vi "Default Instrument Setup.vi"(8 "error in (no error)":errorcluster, 11 "VISA resource name":refnum<visa-resource-name>) -> (0 "error out":errorcluster, 3 "VISA resource name out":refnum<visa-resource-name>)   [LabVIEW 2013, in "Tektronix DPO MSO 2000 4000 Series.lvlib"]
doc: "This Utility VI sends a default command string to the instrument whenever a new VISA session is opened, or the instrument is reset. Use this VI as a subVI for the <B>Initialize</B> and <B>Reset</B> VIs. Altering this VI could cause these two VIs to operate incorrectly."
uses:
  Tektronix DPO MSO 2000 4000 Series.lvlib
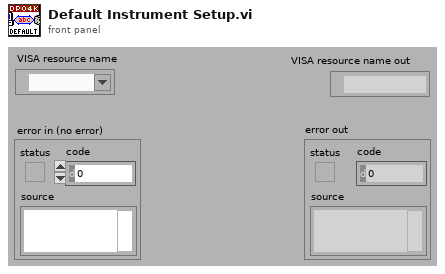
[diagram p1: front panel]
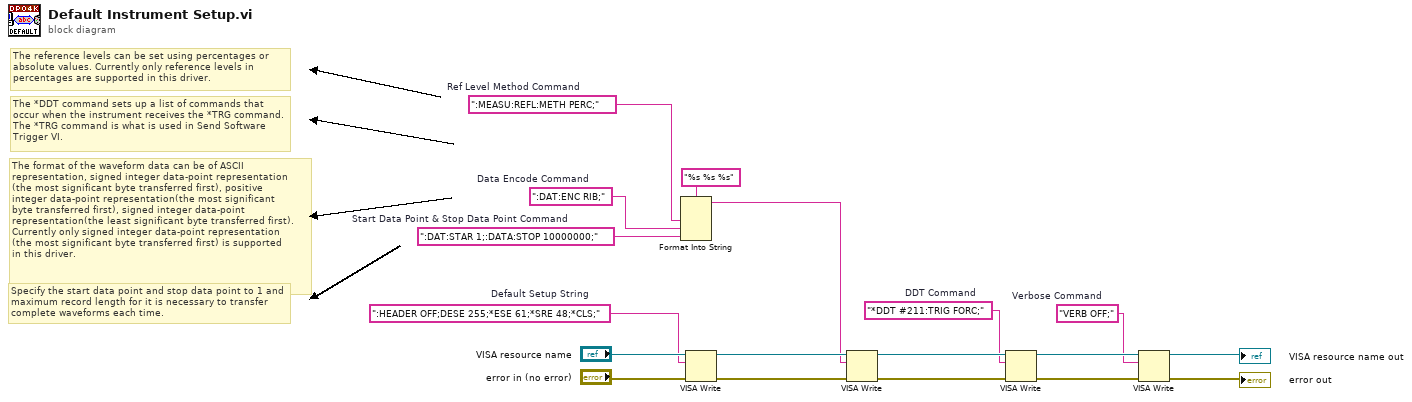
[diagram p0: block diagram]
diagram:
  w1 = "VERB OFF;"  # Verbose Command
  w6 = "*DDT #211:TRIG FORC;"  # DDT Command
  w10 = ":DAT:ENC RIB;"  # Data Encode Command
  w15 = ":MEASU:REFL:METH PERC;"  # Ref Level Method Command
  w9 = ":DAT:STAR 1;:DATA:STOP 10000000;"  # Start Data Point & Stop Data Point Command
  w16 = ":HEADER OFF;DESE 255;*ESE 61;*SRE 48;*CLS;"  # Default Setup String
  # "Specify the start data point and stop data point to 1 and maximum record length for it is necessary to transfer complete waveforms each time."
  # "The format of the waveform data can be of ASCII\nrepresentation, signed integer data-point representation\n(the most significant byte transferred first), positive \ninteger data-point representation(the most significant \nbyte transferred first), signed integer data-point \nrepresentation(the least significant byte transferred first).\nCurrently only signed integer data-point representation\n(the most significant byte transferred first) is supported\nin this driver."
  # "The reference levels can be set using percentages or absolute values. Currently only reference levels in \npercentages are supported in this driver."
  # "The *DDT command sets up a list of commands that occur when the instrument receives the *TRG command.  \nThe *TRG command is what is used in Send Software Trigger VI."
  n1 = Format Into String(format string="%s %s %s", w15, w10, w9) -> (resulting string=w12:string)  [unwired: 2 in, 1 out]
  n2 = VISA Write(VISA resource name="VISA resource name", write buffer=w16, error in (no error)="error in (no error)") -> (VISA resource name out=w14:refnum<visa-resource-name>, error out=w13:errorcluster)  [unwired: 1 out]
  n3 = VISA Write(VISA resource name=w14, write buffer=w12, error in (no error)=w13) -> (VISA resource name out=w8:refnum<visa-resource-name>, error out=w7:errorcluster)  [unwired: 1 out]
  n4 = VISA Write(VISA resource name=w8, write buffer=w6, error in (no error)=w7) -> (VISA resource name out=w5:refnum<visa-resource-name>, error out=w4:errorcluster)  [unwired: 1 out]
  n5 = VISA Write(VISA resource name=w5, write buffer=w1, error in (no error)=w4) -> (VISA resource name out=→"VISA resource name out":refnum<visa-resource-name>, error out=→"error out":errorcluster)  [unwired: 1 out]
